vi "Temperature Out of Range.vi"(2 "Temperature":dbl, 3 "Lower Limit":dbl, 4 "Upper Limit":dbl, 5 "error in (no error)":errorcluster) -> (18 "Out Of Range":bool, 19 "error out":errorcluster)   [LabVIEW 2017, in "Temp.lvclass"]
uses:
  Temp.lvclass
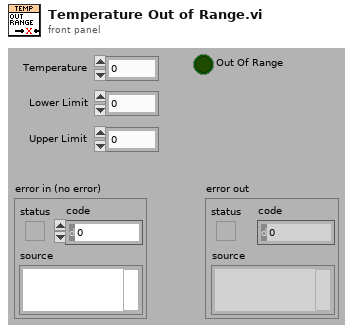
[diagram p1: front panel]
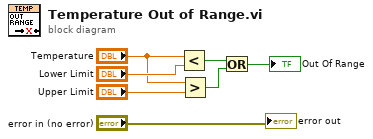
[diagram p0: block diagram]
diagram:
  n1 = Less?(x="Temperature", y="Lower Limit") -> (x < y?=w2:bool)
  n2 = Greater?(x="Temperature", y="Upper Limit") -> (0:w1:bool)
  n3 = Or(x=w2, y=w1) -> (x .or. y?=→"Out Of Range":bool)
  "error out" <- "error in (no error)"
